vi "Init_Data_array.vi"() -> (0 "Data Cluster":T1)   [LabVIEW 2015]
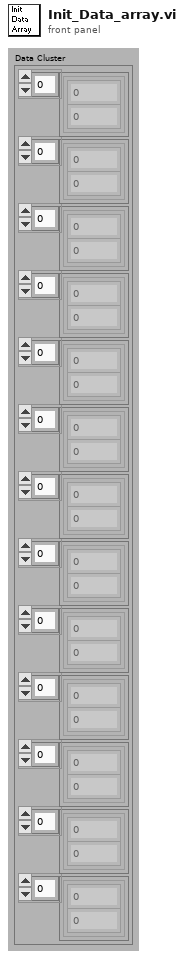
[diagram p1: front panel]
types:
  T1 = cluster{cluster{sgl, sgl}[], cluster{sgl, sgl}[], cluster{sgl, sgl}[], cluster{sgl, sgl}[], cluster{sgl, sgl}[], cluster{sgl, sgl}[], cluster{sgl, sgl}[], cluster{sgl, sgl}[], cluster{sgl, sgl}[], cluster{sgl, sgl}[], cluster{sgl, sgl}[], cluster{sgl, sgl}[], cluster{sgl, sgl}[]}
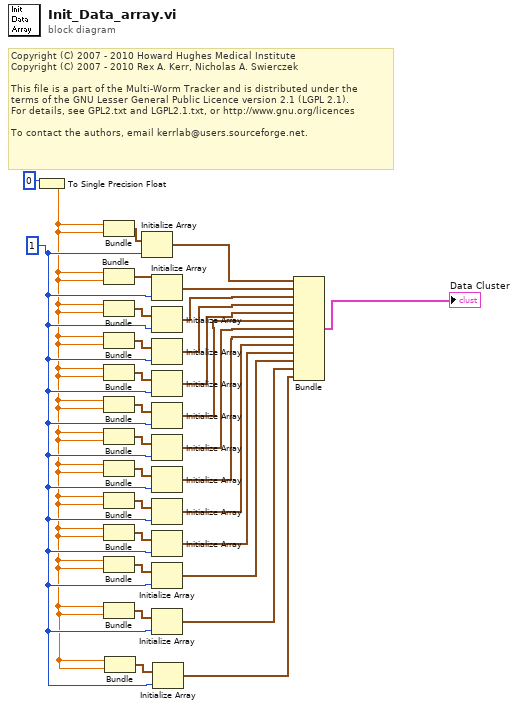
[diagram p0: block diagram]
diagram:
  w3 = 1 ("dimension size")
  # "Copyright (C) 2007 - 2010 Howard Hughes Medical Institute\nCopyright (C) 2007 - 2010 Rex A. Kerr, Nicholas A. Swierczek\n \nThis file is a part of the Multi-Worm Tracker and is distributed under the\nterms of the GNU Lesser General Public Licence version 2.1 (LGPL 2.1).\nFor details, see GPL2.txt and LGPL2.1.txt, or http://www.gnu.org/licences\n \nTo contact the authors, email kerrlab@users.sourceforge.net."
  n1 = To Single Precision Float(number=0) -> (single precision float=w2:sgl)
  n2 = Bundle(w2, w2) -> (w27:cluster{sgl, sgl})  [unwired: 1 in]
  n3 = Bundle(w2, w2) -> (w28:cluster{sgl, sgl})  [unwired: 1 in]
  n4 = Bundle(w2, w2) -> (w25:cluster{sgl, sgl})  [unwired: 1 in]
  n5 = Bundle(w2, w2) -> (w24:cluster{sgl, sgl})  [unwired: 1 in]
  n6 = Bundle(w2, w2) -> (w23:cluster{sgl, sgl})  [unwired: 1 in]
  n7 = Bundle(w2, w2) -> (w22:cluster{sgl, sgl})  [unwired: 1 in]
  n8 = Bundle(w2, w2) -> (w21:cluster{sgl, sgl})  [unwired: 1 in]
  n9 = Bundle(w2, w2) -> (w20:cluster{sgl, sgl})  [unwired: 1 in]
  n10 = Bundle(w2, w2) -> (w19:cluster{sgl, sgl})  [unwired: 1 in]
  n11 = Bundle(w2, w2) -> (w18:cluster{sgl, sgl})  [unwired: 1 in]
  n12 = Bundle(w2, w2) -> (w17:cluster{sgl, sgl})  [unwired: 1 in]
  n13 = Bundle(w2, w2) -> (w6:cluster{sgl, sgl})  [unwired: 1 in]
  n14 = Bundle(w2, w2) -> (w4:cluster{sgl, sgl})  [unwired: 1 in]
  n15 = Initialize Array(w27, w3) -> (w30:cluster{sgl, sgl}[])
  n16 = Initialize Array(w28, w3) -> (w29:cluster{sgl, sgl}[])
  n17 = Initialize Array(w25, w3) -> (w16:cluster{sgl, sgl}[])
  n18 = Initialize Array(w24, w3) -> (w15:cluster{sgl, sgl}[])
  n19 = Initialize Array(w23, w3) -> (w14:cluster{sgl, sgl}[])
  n20 = Initialize Array(w22, w3) -> (w13:cluster{sgl, sgl}[])
  n21 = Initialize Array(w21, w3) -> (w12:cluster{sgl, sgl}[])
  n22 = Initialize Array(w20, w3) -> (w11:cluster{sgl, sgl}[])
  n23 = Initialize Array(w19, w3) -> (w10:cluster{sgl, sgl}[])
  n24 = Initialize Array(w18, w3) -> (w9:cluster{sgl, sgl}[])
  n25 = Initialize Array(w17, w3) -> (w8:cluster{sgl, sgl}[])
  n26 = Initialize Array(w6, w3) -> (w5:cluster{sgl, sgl}[])
  n27 = Initialize Array(w4, w3) -> (w1:cluster{sgl, sgl}[])
  n28 = Bundle(w30, w29, w16, w15, w14, w13, w12, w11, w10, w9, w8, w5, w1) -> (→"Data Cluster":T1)  [unwired: 1 in]
